vi "num analysis.vi"(0 "x":i32) -> (1 "Color":i32, 2 "Chess":i32, 3 "Num":i32)   [LabVIEW 2009]
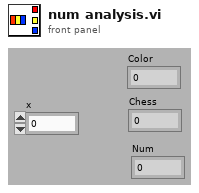
[diagram p1: front panel]
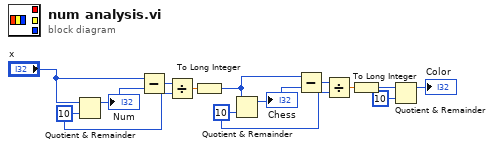
[diagram p0: block diagram]
diagram:
  w10 = 10 ("y")
  w11 = 10 ("y")
  n1 = Quotient & Remainder(x="x", y=w11) -> (x-y*floor(x/y)=w13:i32)  [unwired: 1 out]
  "Num" <- w13
  n2 = Subtract(x="x", y=w13) -> (x-y=w12:i32)
  n3 = Divide(x=w12, y=w11) -> (x/y=w8:dbl)
  n4 = To Long Integer(number=w8) -> (32bit integer=w6:i32)
  n5 = Quotient & Remainder(x=w6, y=w10) -> (x-y*floor(x/y)=w9:i32)  [unwired: 1 out]
  "Chess" <- w9
  n6 = Subtract(x=w6, y=w9) -> (x-y=w7:i32)
  n7 = Divide(x=w7, y=w10) -> (x/y=w4:dbl)
  n8 = To Long Integer(number=w4) -> (32bit integer=w3:i32)
  n9 = Quotient & Remainder(x=w3, y=10) -> (x-y*floor(x/y)=→"Color":i32)  [unwired: 1 out]
